vi "Count Matched testCases.vi"(7 "test":T1, 9 "Total":u32, 11 "Matrix":bool[][](array[boolean])) -> (0 "Pct":dbl, 2 "Nb Test Cases":u32)   [LabVIEW 2021, in "Bananas.lvlib" / "Pips.lvclass"]
uses:
  Pips.lvclass
  row_col_test -- enum.ctl
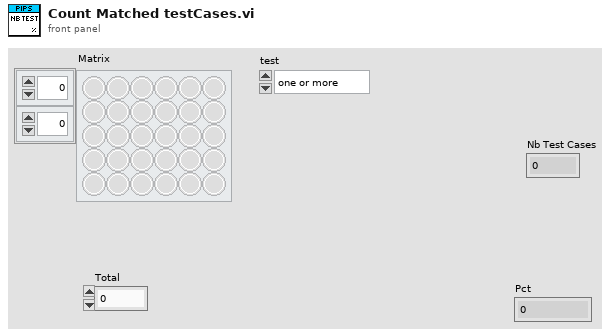
[diagram p1: front panel]
types:
  T1 = typedef "Bananas.lvlib/Pips.lvclass/row_col_test -- enum.ctl" = enum16{"one or more", "all", "none"}
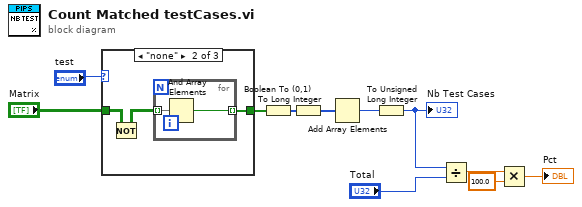
[diagram p0: block diagram]
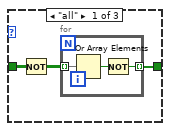
[diagram p2: hidden frame]
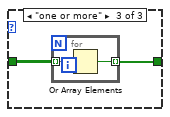
[diagram p3: hidden frame]
diagram:
  n1 = case shown="\"none\"" "test" {
    tunnel: [w14 w20 w24] -> w7
    tunnel: "Matrix" -> [w13 w18 w23]
    frame "all" {
      n2 = Not(x=w13) -> (.not. x?=w12:bool[][])
      n3 = for {
        tunnel: w12 -> [w17] mode=indexing
        tunnel: [w15] -> w14 mode=indexing
        n4 = Or Array Elements(Boolean array=w17) -> (logical OR=w16:bool)
        n5 = Not(x=w16) -> (.not. x?=w15:bool)
      }
    }
    frame "none" {
      n6 = Not(x=w18) -> (.not. x?=w19:bool[][])
      n7 = for {
        tunnel: w19 -> [w22] mode=indexing
        tunnel: [w21] -> w20 mode=indexing
        n8 = And Array Elements(Boolean array=w22) -> (logical AND=w21:bool)
      }
    }
    frame "one or more" {
      n9 = for {
        tunnel: w23 -> [w26] mode=indexing
        tunnel: [w25] -> w24 mode=indexing
        n10 = Or Array Elements(Boolean array=w26) -> (logical OR=w25:bool)
      }
    }
  }
  n11 = Boolean To (0,1)(Boolean=w7) -> (0, 1=w9:i16[])
  n12 = To Long Integer(number=w9) -> (32bit integer=w10:i32[])
  n13 = Add Array Elements(numeric array=w10) -> (sum=w11:i32)
  n14 = To Unsigned Long Integer(number=w11) -> (unsigned 32bit integer=w1:u32)
  "Nb Test Cases" <- w1
  n15 = Divide(x=w1, y="Total") -> (x/y=w5:dbl)
  n16 = Multiply(x=w5, y=100.0) -> (x*y=→"Pct":dbl)
